vi "Read Group.vi"(8 "error in (no error)":errorcluster, 10 "Group ID":string, 11 "dsf refnum":T1) -> (0 "error out":errorcluster, 1 "value":T2, 3 "dsf refnum out":T1, 4 "found?":bool)   [LabVIEW 2017, in "Data Sharing Framework Configuration.lvlib"]
doc: "Reads a value associated with a key in a specified section from the configuration data identified by <B>dsf refnum</B>. If the key does not exist, the VI returns the default value. This VI supports multibyte characters in strings. Wire data to the <B>default value</B> input to determine the polymorphic instance to use or manually select the instance."
uses:
  Data Sharing Framework Configuration.lvlib
  Controls/DSF Group Info.ctl
  Controls/DSF Direction.ctl
  Controls/DSF Timing Info.ctl
  Controls/DSF Config Data RefNum.ctl
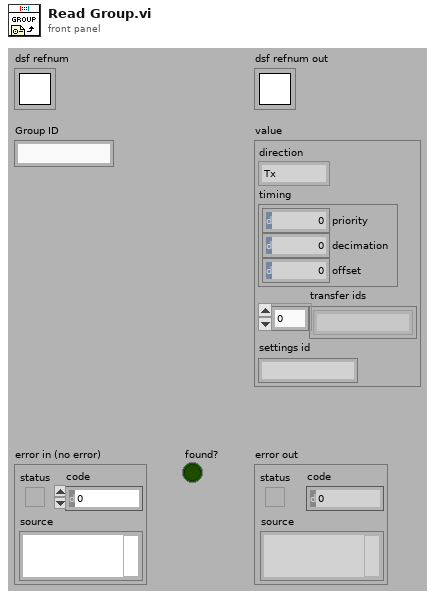
[diagram p1: front panel]
types:
  T1 = typedef "Data Sharing Framework Configuration.lvlib/DSF Config Data RefNum.ctl" = refnum<k1>
  T2 = typedef "Data Sharing Framework Configuration.lvlib/DSF Group Info.ctl" = cluster{"direction":T3, "timing":T4, "transfer ids":string[], "settings id":string}
  T3 = typedef "Data Sharing Framework Configuration.lvlib/DSF Direction.ctl" = enum8{"Tx", "Rx"}
  T4 = typedef "Data Sharing Framework Configuration.lvlib/DSF Timing Info.ctl" = cluster{"priority":u64, "decimation":u64, "offset":u64}
  T5 = typedef "Data Sharing Framework Configuration.lvlib/DSF Configuration Reference.ctl" = refnum<data-value>
  T6 = typedef "Data Sharing Framework Configuration.lvlib/Internal.DSF Configuration.ctl" = cluster{"dsfversion":T7, "version":T7, "plugins":T8[], "groups":T10[], "transfers":T12[], "channels":T14[], "settings":T16[]}
  T7 = typedef "Data Sharing Framework Configuration.lvlib/DSF Version Info.ctl" = cluster{"major":u32, "minor":u32, "fix":u32, "build":string}
  T8 = typedef "Data Sharing Framework Configuration.lvlib/Internal.DSF Plugin with ID.ctl" = cluster{"id":string, "values":T9}
  T9 = typedef "Data Sharing Framework Configuration.lvlib/Internal.DSF Plugin Info.ctl" = cluster{"type":string, "timing":T4, "group ids":string[], "settings id":string}
  T10 = typedef "Data Sharing Framework Configuration.lvlib/Internal.DSF Group with ID.ctl" = cluster{"id":string, "values":T11}
  T11 = typedef "Data Sharing Framework Configuration.lvlib/Internal.DSF Group Info.ctl" = cluster{"direction":i32, "timing":T4, "transfer ids":string[], "settings id":string}
  T12 = typedef "Data Sharing Framework Configuration.lvlib/Internal.DSF Transfer with ID.ctl" = cluster{"id":string, "values":T13}
  T13 = typedef "Data Sharing Framework Configuration.lvlib/Internal.DSF Transfer Info.ctl" = cluster{"byte order":i32, "channel ids":string[], "settings id":string}
  T14 = typedef "Data Sharing Framework Configuration.lvlib/Internal.DSF Channel with ID.ctl" = cluster{"id":string, "values":T15}
  T15 = typedef "Data Sharing Framework Configuration.lvlib/Internal.DSF Channel Info.ctl" = cluster{"count":u64, "buffer offset":u64, "data type":i32, "settings id":string}
  T16 = typedef "Data Sharing Framework Configuration.lvlib/Internal.DSF Settings with ID.ctl" = cluster{"id":string, "values":T17}
  T17 = typedef "Data Sharing Framework Configuration.lvlib/Internal.DSF Settings Info.ctl" = cluster{"key":string, "value":string}[]
  T18 = cluster{"dsf configuration":T6, "path":path, "dirty":bool}
  T19 = typedef "Data Sharing Framework Configuration.lvlib/DSF Config Data.ctl" = cluster{"dsf configuration":T6, "path":path, "dirty":bool}
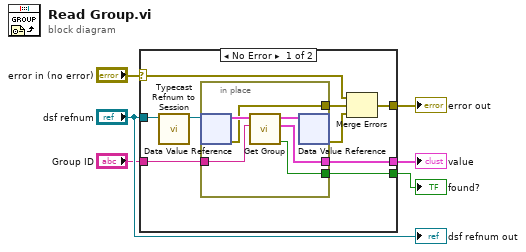
[diagram p0: block diagram]
diagram:
  n1 = case shown="No Error" "error in (no error)" {
    selector: "error in (no error)" -> [w8 w22]
    tunnel: "dsf refnum" -> [w15 _]
    tunnel: [w7 w22] -> w4
    tunnel: "Group ID" -> [w14 _]
    tunnel: [w13 _] -> w2
    tunnel: [w12 _] -> w1
    frame No Error {
      n2 = call "Typecast Refnum to Session.vi"("dsf refnum in"=w15) -> ("DSF Configuration Session out"=w11:T5)  [unwired: 10 in]
      n3 = in-place {
        in-place-border: w14 -> [w21]
        in-place-border: [w20] -> w13
        in-place-border: [w19] -> w12
        in-place-border: [w16] -> w9
        n4 = in-place-dvr #1(w11) -> (w18:T18, w16:errorcluster)
        n5 = call "Get Group.vi"("id"=w21, "DSF Configuration in"=w18) -> ("exists?"=w19:bool, "info"=w20:T2, "DSF Configuration out"=w17:T19)  [unwired: 6 in, 1 out]
        n6 = in-place-dvr #1(w17) -> (w10:errorcluster)  [unwired: 1 out]
      }
      n7 = Merge Errors(w8, w9, w10) -> (w7:errorcluster)
    }
    frame Error {
    }
  }
  "error out" <- w4
  "found?" <- w1
  "value" <- w2
  "dsf refnum out" <- "dsf refnum"
